vi "ZAD2.vi"(6 "Skala":bool, 9 "Precyzja":u8, 10 "Rodzaj czujnika":u8(knob) scale=0.0..1.0, 11 "Numeric in":dbl) -> (2 "Numeric out":dbl, 3 "Error":bool)   [LabVIEW 2017]
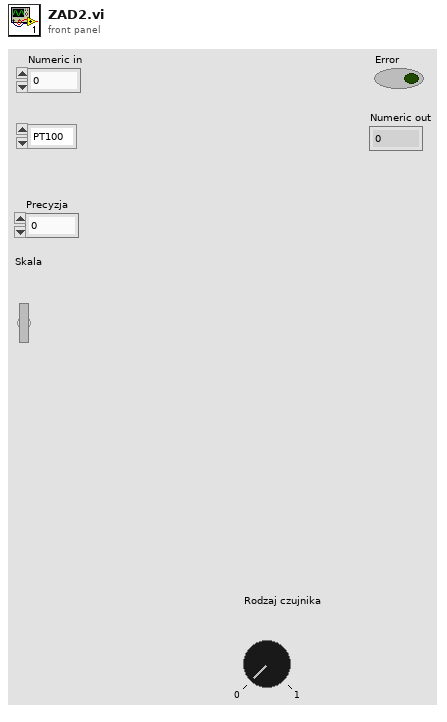
[diagram p1: front panel]
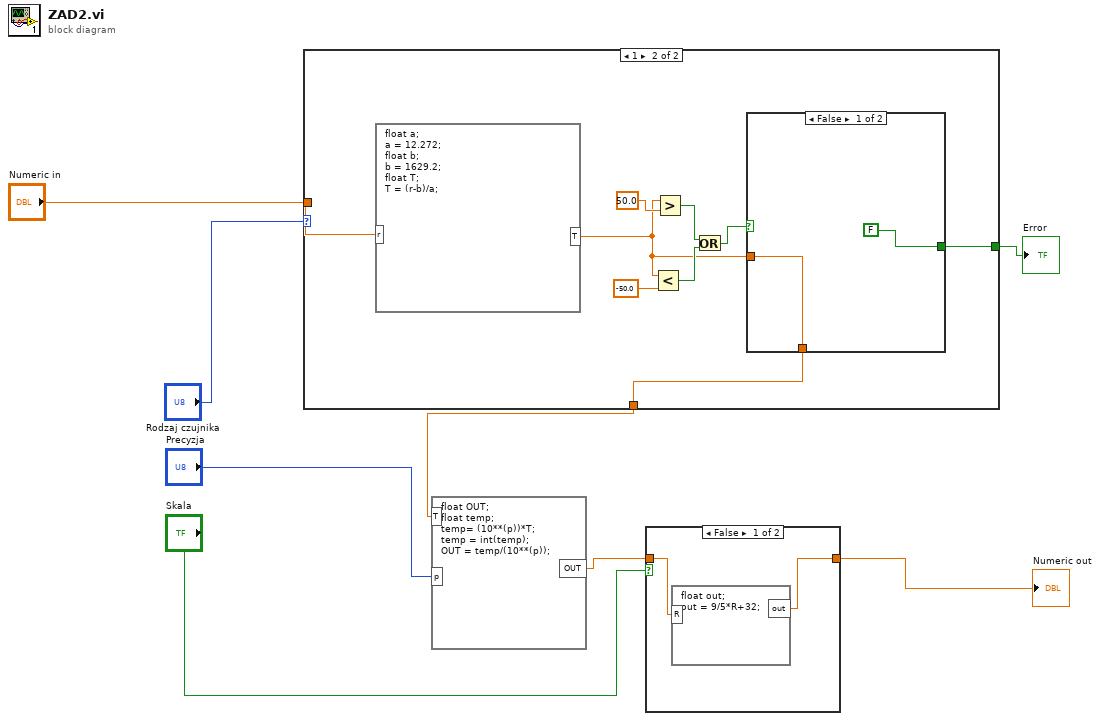
[diagram p0: block diagram]
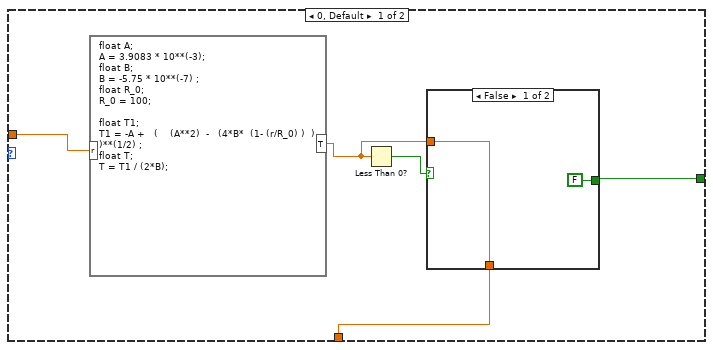
[diagram p3: hidden frame]
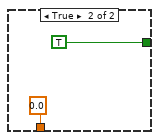
[diagram p4: hidden frame]
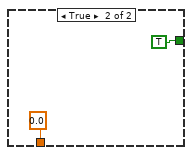
[diagram p5: hidden frame]
diagram:
  n1 = case shown="1" "Rodzaj czujnika" {
    tunnel: "Numeric in" -> [w13 w26]
    tunnel: [w11 w22] -> w4
    tunnel: [w9 w21] -> w8
    frame 0, Default {
      n2 = formula code="float A;\nA = 3.9083 * 10**(-3);\nfloat B;\nB = -5.75 * 10**(-7) ;\nfloat R_0;\nR_0 = 100;\n\nfloat T1;\nT1 = -A +   (    (A**2)  -   (4*B*  (1- (r/R_0) )  )      )**(1/2) ;\nfloat T;  \nT = T1 / (2*B);"("r"=w13) -> ("T"=w10:dbl)
      n3 = Less Than 0?(x=w10) -> (x < 0?=w12:bool)
      n4 = case shown="False" w12 {
        tunnel: [w15 0.0] -> w11
        tunnel: w10 -> [w15 _]
        tunnel: [FALSE ("Error") TRUE ("Error")] -> w9
        frame False {
        }
        frame True {
        }
      }
    }
    frame 1 {
      n5 = formula code="float a;\na = 12.272;\nfloat b;\nb = 1629.2;\nfloat T;\nT = (r-b)/a;"("r"=w26) -> ("T"=w19:dbl)
      n6 = Less?(x=w19, y=-50.0) -> (x < y?=w25:bool)
      n7 = Greater?(x=w19, y=50.0) -> (0:w24:bool)
      n8 = Or(x=w24, y=w25) -> (x .or. y?=w23:bool)
      n9 = case shown="False" w23 {
        tunnel: [w27 0.0] -> w22
        tunnel: w19 -> [w27 _]
        tunnel: [FALSE ("Error") TRUE ("Error")] -> w21
        frame False {
        }
        frame True {
        }
      }
    }
  }
  "Error" <- w8
  n10 = formula code="float OUT;\nfloat temp;\ntemp= (10**(p))*T;\ntemp = int(temp);\nOUT = temp/(10**(p));"("p"="Precyzja", "T"=w4) -> ("OUT"=w7:dbl)
  n11 = case shown="False" "Skala" {
    tunnel: [w31 w33] -> w6
    tunnel: w7 -> [w32 w33]
    frame False {
      n12 = formula code="float out;\nout = 9/5*R+32;"("R"=w32) -> ("out"=w31:dbl)
    }
    frame True {
    }
  }
  "Numeric out" <- w6
